vi "Hash.vi"(11 "String":string) -> (3 "Numeric":u64)   [LabVIEW 2021]
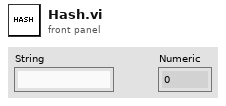
[diagram p1: front panel]
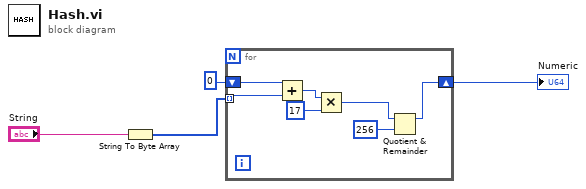
[diagram p0: block diagram]
diagram:
  n1 = String To Byte Array(string="String") -> (unsigned byte array=w1:u8[])
  n2 = for {
    tunnel: w1 -> [w10] mode=indexing
    shift-right: [w5] -> w3
    shift-left: u64 0 -> [w11]
    n3 = Add(x=w11, y=w10) -> (x+y=w9:u64)
    n4 = Multiply(x=w9, y=u64 17) -> (x*y=w7:u64)
    n5 = Quotient & Remainder(x=w7, y=u64 256) -> (x-y*floor(x/y)=w5:u64)  [unwired: 1 out]
  }
  "Numeric" <- w3
